vi "editDefaultAmount.vi"(8 "error in (no error)":errorcluster, 11 "Category in":refnum<class "Category.lvclass">) -> (0 "error out":errorcluster, 2 "UserConfirm?":bool, 3 "Category out":refnum<class "Category.lvclass">)   [LabVIEW 2020, in "Category.lvclass"]
uses:
  Category.lvclass
  UserEditableAmount/UserEditableAmount.lvclass
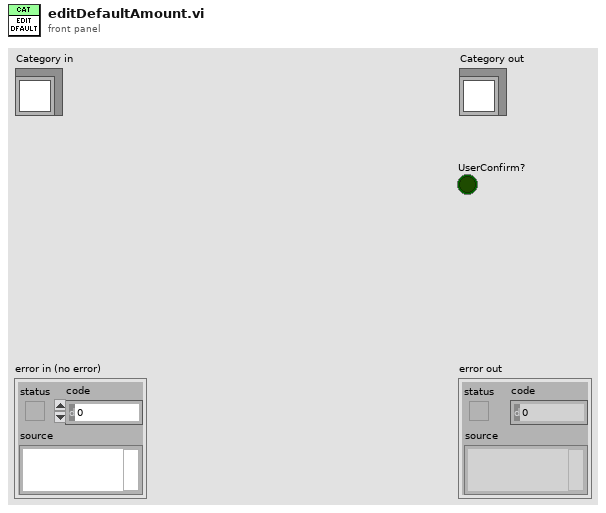
[diagram p1: front panel]
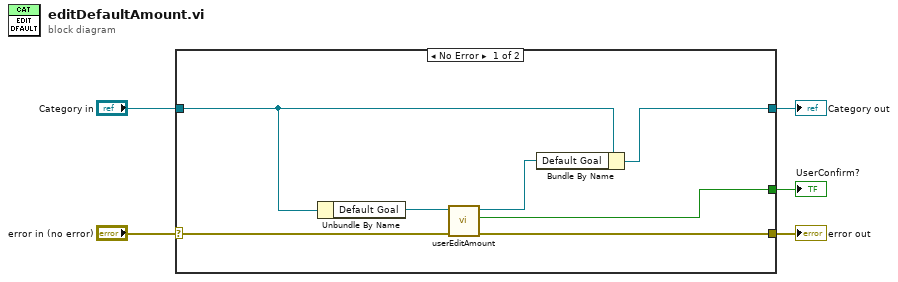
[diagram p0: block diagram]
diagram:
  n1 = case shown="No Error" "error in (no error)" {
    selector: "error in (no error)" -> [w11 w14]
    tunnel: [w10 w14] -> w4
    tunnel: [w7 w13] -> w2
    tunnel: "Category in" -> [w9 w13]
    tunnel: [w6 _] -> w1
    frame No Error {
      n2 = Unbundle By Name(w9) -> ("Default Goal"=w12:refnum<class "UserEditableAmount.lvclass">)
      n3 = call "userEditAmount.vi"("error in (no error)"=w11, "UserEditableAmount.lvclass"=w12) -> ("error out"=w10:errorcluster, "UserConfirm?"=w6:bool, "UserEditableAmount.lvclass"=w8:refnum<class "UserEditableAmount.lvclass">)  [unwired: 7 in]
      n4 = Bundle By Name(cluster=w9, "Default Goal"=w8) -> (w7:refnum<class "Category.lvclass">)
    }
    frame Error {
    }
  }
  "error out" <- w4
  "Category out" <- w2
  "UserConfirm?" <- w1
